vi "Read MessageRefnum.vi"(8 "error in (no error)":errorcluster, 11 "CS++Message in":refnum<class "CS++Message.lvclass">) -> (0 "error out":errorcluster, 2 "MessageRefnum":refnum<vi>, 3 "CS++Message out":refnum<class "CS++Message.lvclass">)   [LabVIEW 2015, in "CS++Message.lvlib" / "CS++Message.lvclass"]
uses:
  CS++Message.lvclass
  CS++Message.lvclass/CS++Message.ctl
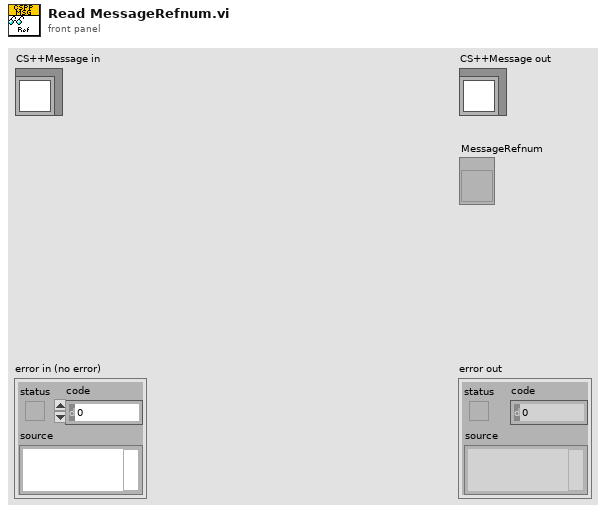
[diagram p1: front panel]
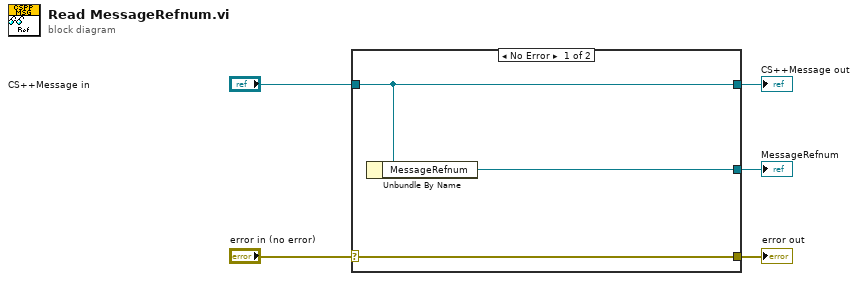
[diagram p0: block diagram]
diagram:
  n1 = case shown="No Error" "error in (no error)" {
    selector: "error in (no error)" -> [w8 w9]
    tunnel: [w8 w9] -> w4
    tunnel: [w7 w10] -> w2
    tunnel: "CS++Message in" -> [w7 w10]
    tunnel: [w6 _] -> w1
    frame No Error {
      n2 = Unbundle By Name(w7) -> ("MessageRefnum"=w6:refnum<vi>)
    }
    frame Error {
    }
  }
  "error out" <- w4
  "CS++Message out" <- w2
  "MessageRefnum" <- w1
